vi "ScanSteuerung_to_Datapoints.vi"(2 "Datapoints (-1=estimate)":i32=-1, 3 "ScanSteuerung":T3(array[cluster])=[{"Zeitpunkt [s]"=0.0, "Wirkung"=enum."Abs", "Kanal"=enum."GalvoX", "Wert (/s)"=0.0}, {"Zeitpunkt [s]"=0.0, "Wirkung"=enum."Abs", "Kanal"=enum."GalvoY", "Wert (/s)"=0.5}, {"Zeitpunkt [s]"=0.0, "Wirkung"=enum."LoopStart", "Kanal"=enum."Loop", "Wert (/s)"=3.0}, {"Zeitpunkt [s]"=0.0, "Wirkung"=enum."LoopStart", "Kanal"=enum."Loop", "Wert (/s)"=2.0}, {"Zeitpunkt [s]"=0.0, "Wirkung"=enum."Inc", "Kanal"=enum."GalvoX", "Wert (/s)"=10.0}, {"Zeitpunkt [s]"=0.0, "Wirkung"=enum."IncInc", "Kanal"=enum."GalvoX", "Wert (/s)"=-100.0}, {"Zeitpunkt [s]"=0.0, "Wirkung"=enum."IncInc", "Kanal"=enum."GalvoY", "Wert (/s)"=-100.0}, {"Zeitpunkt [s]"=0.1, "Wirkung"=enum."IncInc", "Kanal"=enum."GalvoY", "Wert (/s)"=100.0}, {"Zeitpunkt [s]"=0.2, "Wirkung"=enum."IncInc", "Kanal"=enum."GalvoX", "Wert (/s)"=100.0}, {"Zeitpunkt [s]"=0.3, "Wirkung"=enum."IncInc", "Kanal"=enum."GalvoY", "Wert (/s)"=-100.0}, {"Zeitpunkt [s]"=0.4, "Wirkung"=enum."IncInc", "Kanal"=enum."GalvoX", "Wert (/s)"=0.0}, {"Zeitpunkt [s]"=0.4, "Wirkung"=enum."LoopEnd", "Kanal"=enum."Loop", "Wert (/s)"=0.0}, {"Zeitpunkt [s]"=0.802, "Wirkung"=enum."LoopEnd", "Kanal"=enum."Loop", "Wert (/s)"=0.0}, {"Zeitpunkt [s]"=2.5, "Wirkung"=enum."IncInc", "Kanal"=enum."GalvoX", "Wert (/s)"=0.0}], 4 "Aktiv":T2(array[ring])=[enum."GalvoX", enum."GalvoY"], 5 "Neues Zeitraster":dbl=1e-05) -> (0 "ScanSteuerungOut":T1(array[cluster])=[{"Zeitpunkt [s]"=0.0, "Wirkung"=enum."Abs", "Kanal"=0.0, "Wert (/s)"=0.0}, {"Zeitpunkt [s]"=0.0, "Wirkung"=enum."Inc", "Kanal"=0.0, "Wert (/s)"=0.0001}, {"Zeitpunkt [s]"=0.0, "Wirkung"=enum."Abs", "Kanal"=1.0, "Wert (/s)"=0.5}, {"Zeitpunkt [s]"=0.0, "Wirkung"=enum."IncInc", "Kanal"=0.0, "Wert (/s)"=-1.0000000000000002e-08}, {"Zeitpunkt [s]"=0.0, "Wirkung"=enum."IncInc", "Kanal"=1.0, "Wert (/s)"=-1.0000000000000002e-08}, {"Zeitpunkt [s]"=10000.0, "Wirkung"=enum."IncInc", "Kanal"=1.0, "Wert (/s)"=1.0000000000000002e-08}, {"Zeitpunkt [s]"=20000.0, "Wirkung"=enum."IncInc", "Kanal"=0.0, "Wert (/s)"=1.0000000000000002e-08}, {"Zeitpunkt [s]"=29999.999999999996, "Wirkung"=enum."IncInc", "Kanal"=1.0, "Wert (/s)"=-1.0000000000000002e-08}, {"Zeitpunkt [s]"=40000.0, "Wirkung"=enum."IncInc", "Kanal"=0.0, "Wert (/s)"=0.0}], 1 "Waveform Graph":dbl[][](graph))   [LabVIEW 2011]
panel:
  out "Datapoints":i32=40001
  out "XY Graph":cluster{dbl[], dbl[]}(graph)
  # "After the loop there has to be at lest one datapoint in one activ channel\nOrder: add abs and rel-values, generate pint, add inc, add incinc to inc\ne.g. at t there is inc: t+1 there is the second pont (t,t+1) with one inc!"
  # "now with incinc support!\nnow with nested loops support!"
  # "Missing error handling for wrong loops!"
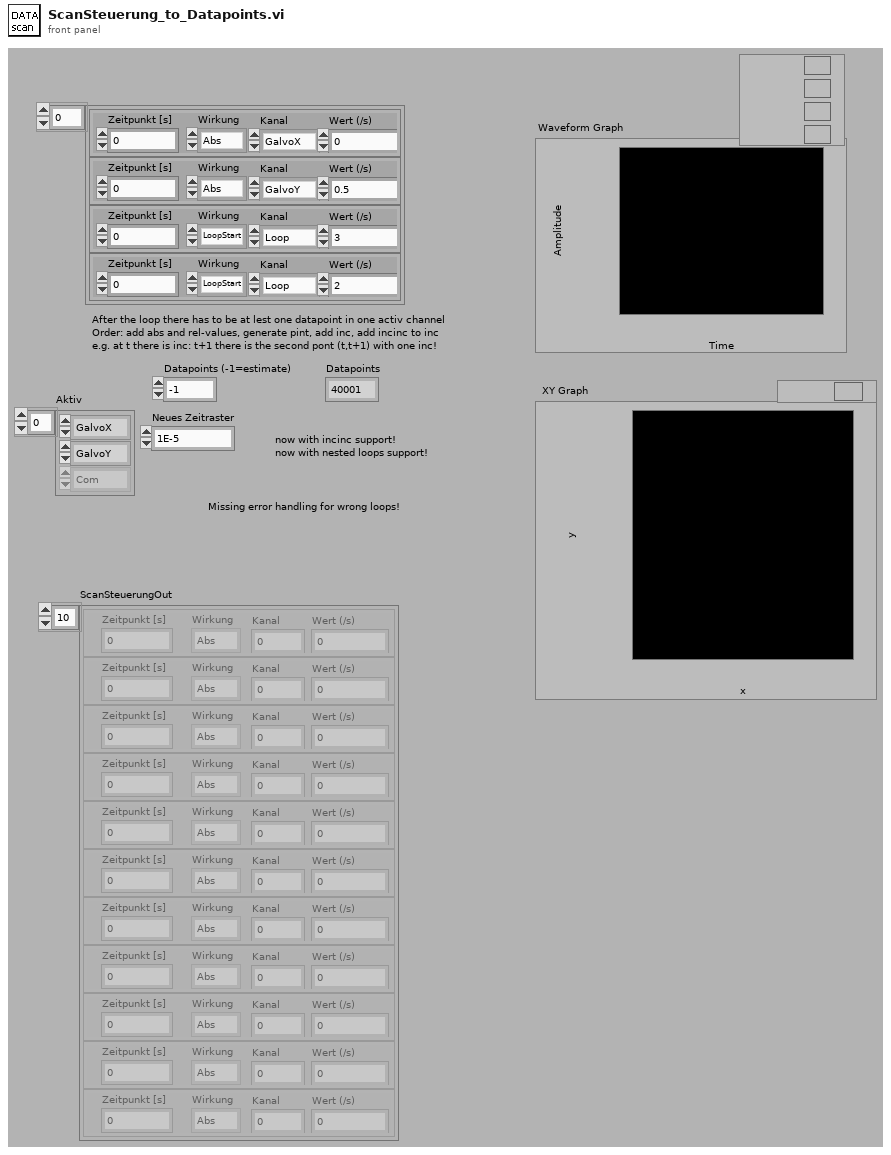
[diagram p1: front panel]
types:
  T1 = cluster{"Zeitpunkt [s]":dbl, "Wirkung":enum16{"Abs", "Rel", "Inc", "IncInc", "LoopStart", "LoopEnd"}, "Kanal":dbl, "Wert (/s)":dbl}[]
  T2 = enum16{"Com", "AnalogConfig", "AnalogValue", "GalvoX", "GalvoY", "Galvo3", "Galvo4", "Digital", "Free", "Loop", "SMoveTime", "Image1X", "Image1Y", "Image2X", "Image2Y"}[]
  T3 = cluster{"Zeitpunkt [s]":dbl, "Wirkung":enum16{"Abs", "Rel", "Inc", "IncInc", "LoopStart", "LoopEnd"}, "Kanal":enum16{"Com", "AnalogConfig", "AnalogValue", "GalvoX", "GalvoY", "Galvo3", "Galvo4", "Digital", "Free", "Loop", "SMoveTime", "Image1X", "Image1Y", "Image2X", "Image2Y"}, "Wert (/s)":dbl}[]
  T4 = cluster{"Time offsets":i32[], "Array":cluster{"Loopstart#":u32, "Loops to do":i32}[]}
  T5 = typedef "ScanControl.ctl" = cluster{"Time [s]":dbl, "action":T6, "channel":T7, "value (/s)":dbl}[]
  T6 = typedef "ScanControl_Action.ctl" = enum16{"Abs", "Rel", "Inc", "IncInc", "LoopStart", "LoopEnd", "WaitTriggerRising"}
  T7 = typedef "ScanControl_Channel.ctl" = enum16{"Com", "AnalogConfig", "AnalogValue", "GalvoX", "GalvoY", "Galvo3", "Galvo4", "Digital", "Free", "Loop", "SMoveTime", "Image1X", "Image1Y", "Image2X", "Image2Y"}
  T8 = cluster{"Zeitpunkt [s]":dbl, "Wirkung":enum16{"Abs", "Rel", "Inc", "IncInc", "LoopStart", "LoopEnd"}, "Kanal":i32, "Wert (/s)":dbl}[]
  T9 = cluster{"Zeitpunkt [s]":dbl, "Wirkung":enum16{"Abs", "Rel", "Inc", "IncInc", "LoopStart", "LoopEnd"}, "Kanal":i32, "Wert (/s)":dbl}
  T10 = enum16{"Abs", "Rel", "Inc", "IncInc", "LoopStart", "LoopEnd"}
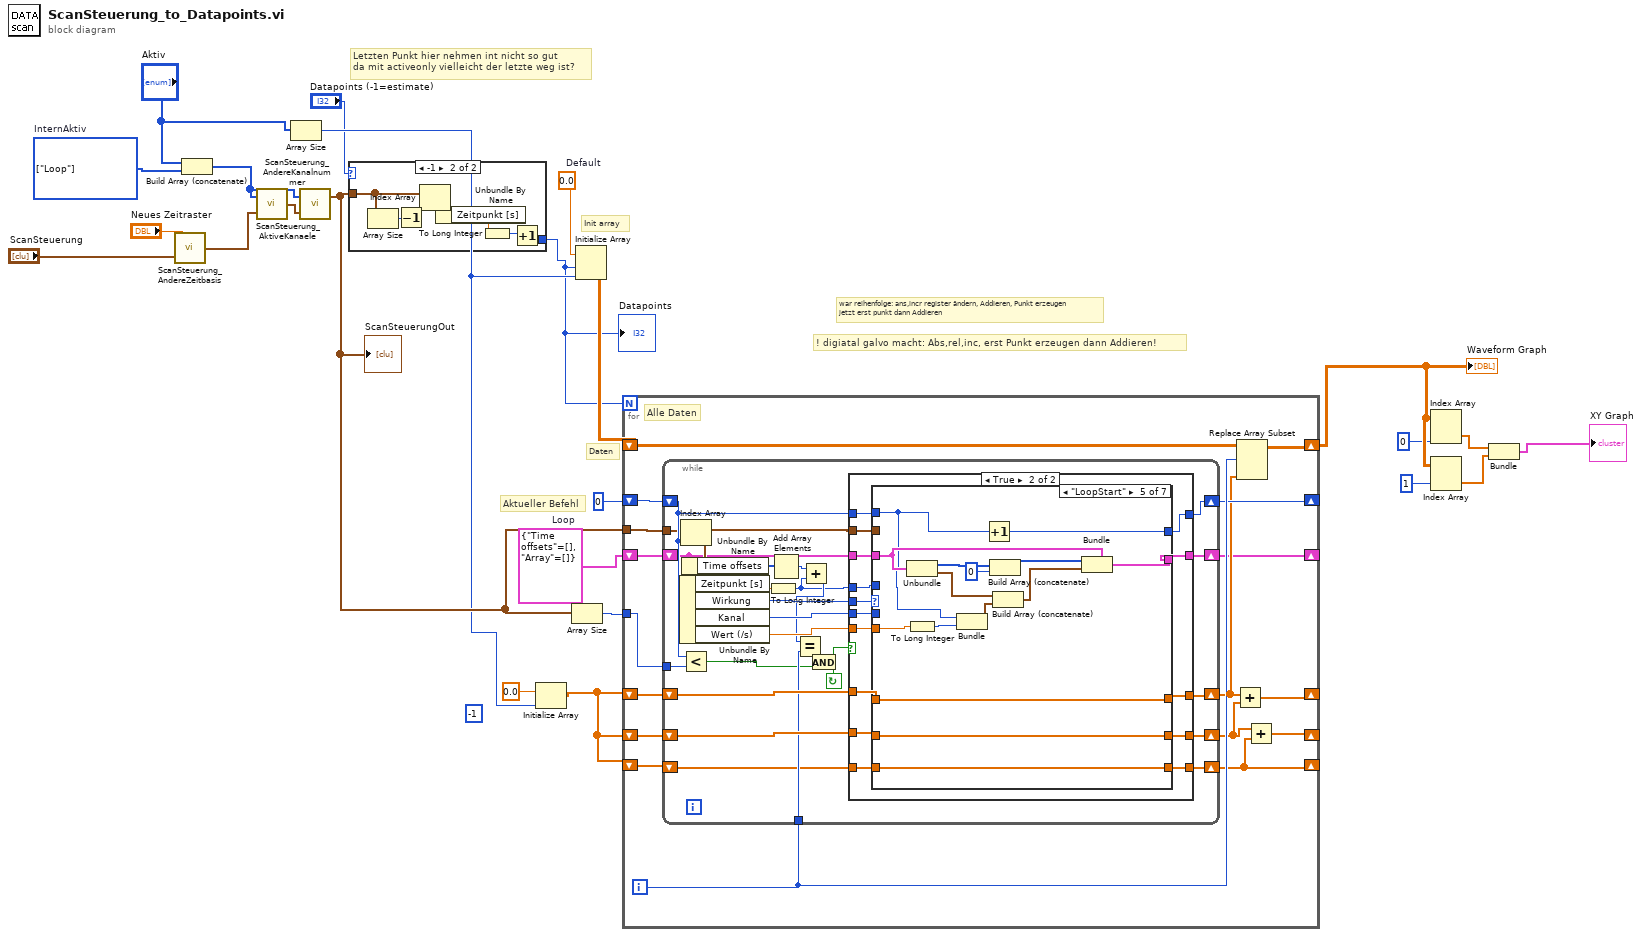
[diagram p0: block diagram]
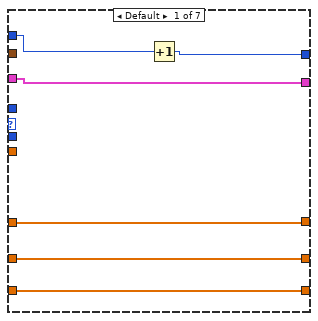
[diagram p4: hidden frame]
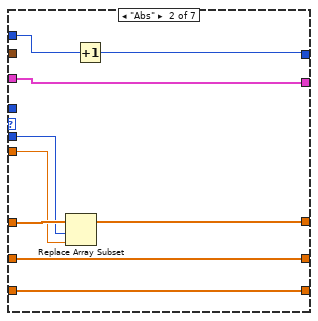
[diagram p5: hidden frame]
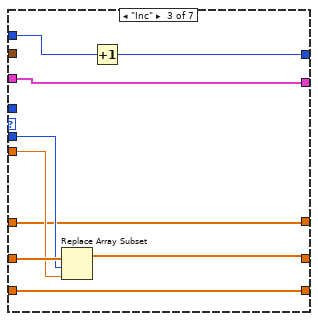
[diagram p6: hidden frame]
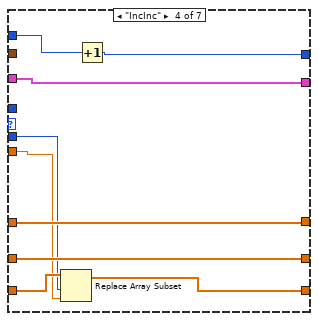
[diagram p7: hidden frame]
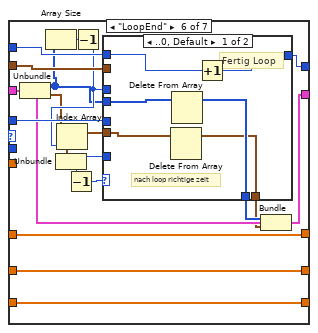
[diagram p8: hidden frame]
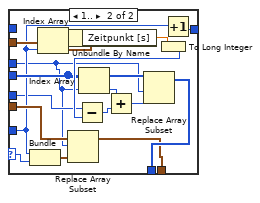
[diagram p9: hidden frame]
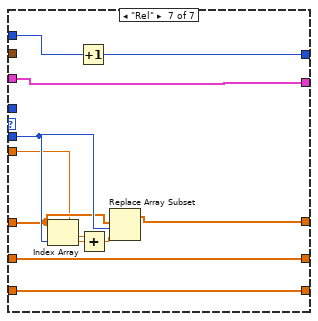
[diagram p10: hidden frame]
diagram:
  (unwired) -1 ("LoopLevel")
  w1 = T4 {"Time offsets"=[], "Array"=[]}  # Loop
  w17 = T2 [enum."Loop"] items=["Com", "AnalogConfig", "AnalogValue", "GalvoX", "GalvoY", "Galvo3", "Galvo4", "Digital", "Free", "Loop", "SMoveTime", "Image1X", "Image1Y", "Image2X", "Image2Y"]  # InternAktiv
  w24 = 0.0  # Default
  # "! digiatal galvo macht: Abs,rel,inc, erst Punkt erzeugen dann Addieren!"
  # "war reihenfolge: ans,incr register ändern, Addieren, Punkt erzeugen\njetzt erst punkt dann Addieren"
  # "Letzten Punkt hier nehmen int nicht so gut\nda mit activeonly vielleicht der letzte weg ist?"
  # "Aktueller Befehl"
  # "Daten"
  # "Init array"
  n1 = call "ScanSteuerung_AndereZeitbasis.vi"("ScanSteuerung"="ScanSteuerung", "Neues Zeitraster"="Neues Zeitraster") -> ("ScanSteuerungOut"=w13:T5)
  n2 = Build Array (concatenate)("Aktiv", w17) -> (w15:T2)
  n3 = call "ScanSteuerung_AktiveKanaele.vi"("ScanSteuerung"=w13, "Aktiv"=w15) -> ("ScanSteuerungOut"=w19:T5)
  n4 = Array Size(array="Aktiv") -> (size(s)=w14:i32)
  n5 = call "ScanSteuerung_AndereKanalnummer.vi"("ScanSteuerung"=w19, "Neue Kanalnummer (nicht gefunden gibt 0!)"=w15) -> ("ScanSteuerungOut"=w18:T8)  [unwired: 1 out]
  "ScanSteuerungOut" <- w18
  n6 = case shown="-1" "Datapoints (-1=estimate)" {
    selector: "Datapoints (-1=estimate)" -> [w25 _]
    tunnel: w18 -> [_ w28]
    tunnel: [w25 w26] -> w4
    frame 0, Default {
    }
    frame -1 {
      n7 = Array Size(array=w28) -> (size(s)=w32:i32)
      n8 = Decrement(x=w32) -> (x-1=w31:i32)
      n9 = Index Array(array=w28, index=w31) -> (element=w30:T9)
      n10 = Unbundle By Name(w30) -> ("Zeitpunkt [s]"=w29:dbl)
      n11 = To Long Integer(number=w29) -> (32bit integer=w27:i32)
      n12 = Increment(x=w27) -> (x+1=w26:i32)
    }
  }
  "Datapoints" <- w4
  n13 = Initialize Array(0.0 ("element"), w14) -> (w2:dbl[])
  n14 = Array Size(array=w18) -> (size(s)=w21:i32)
  n15 = Initialize Array(w24, w4, w14) -> (w22:dbl[][])
  n16 = for {
    N: w4 -> [_]
    shift-left: w2 -> [w47]
    shift-right: [w43] -> _
    tunnel: w21 -> [w40]
    shift-left: u32 0 -> [w48]
    shift-right: [w41] -> _
    shift-left: w22 -> [w45]
    shift-right: [w44] -> w11
    tunnel: w18 -> [w49]
    shift-right: [w37] -> _
    shift-left: w2 -> [w46]
    shift-right: [w35] -> _
    shift-left: w2 -> [w38]
    shift-right: [w33] -> _
    shift-left: w1 -> [w34]
    i -> [w42]
    # "Alle Daten"
    n17 = while {
      tunnel: w49 -> [w54]
      shift-right: [w66] -> w41
      shift-left: w48 -> [w61]
      shift-right: [w69] -> w39
      shift-left: w47 -> [w73]
      shift-right: [w68] -> w36
      shift-left: w46 -> [w72]
      tunnel: w42 -> [w65]
      tunnel: w40 -> [w60]
      shift-right: [w55] -> w35
      shift-left: w38 -> [w56]
      shift-right: [w52] -> w33
      shift-left: w34 -> [w53]
      stop <- w57 continue-if-true
      n18 = Index Array(array=w54, index=w61) -> (element=w74:T9)
      n19 = Unbundle By Name(w74) -> ("Zeitpunkt [s]"=w63:dbl, "Wirkung"=w67:T10, "Kanal"=w71:i32, "Wert (/s)"=w70:dbl)
      n20 = Less?(x=w61, y=w60) -> (x < y?=w58:bool)
      n21 = Unbundle By Name(w53) -> ("Time offsets"=w51:i32[])
      n22 = To Long Integer(number=w63) -> (32bit integer=w62:i32)
      n23 = Add Array Elements(numeric array=w51) -> (sum=w50:i32)
      n24 = Add(x=w50, y=w62) -> (x+y=w64:i32)
      n25 = Equal?(x=w64, y=w65) -> (x = y?=w59:bool)
      n26 = And(x=w59, y=w58) -> (x .and. y?=w57:bool)
      n27 = case shown="True" w57 {
        tunnel: w73 -> [w79 w94]
        tunnel: w72 -> [w78 w93]
        tunnel: w71 -> [_ w92]
        tunnel: w70 -> [_ w91]
        tunnel: [w79 w90] -> w69
        tunnel: [w78 w89] -> w68
        tunnel: w67 -> [_ w88]
        tunnel: w61 -> [w77 w87]
        tunnel: [w77 w86] -> w66
        tunnel: w62 -> [_ w85]
        tunnel: w56 -> [w76 w84]
        tunnel: [w76 w83] -> w55
        tunnel: w54 -> [_ w82]
        tunnel: w53 -> [w75 w81]
        tunnel: [w75 w80] -> w52
        frame False {
          # "Fertig"
        }
        frame True {
          n28 = case shown="\"LoopStart\"" w88 {
            tunnel: w94 -> [w98 w109 w114 w127 w142 w161 w192]
            tunnel: w93 -> [w97 w105 w118 w126 w141 w160 w191]
            tunnel: w92 -> [_ w108 w116 w122 _ _ w193]
            tunnel: w91 -> [_ w107 w115 w121 w140 _ w190]
            tunnel: [w98 w106 w114 w127 w142 w161 w195] -> w90
            tunnel: [w97 w105 w117 w126 w141 w160 w191] -> w89
            tunnel: w87 -> [w100 w104 w113 w125 w135 w158 w188]
            tunnel: [w95 w103 w112 w124 w139 w159 w187] -> w86
            tunnel: w85 -> [_ _ _ _ _ w157 _]
            tunnel: w84 -> [w96 w102 w111 w123 w138 w156 w186]
            tunnel: [w96 w102 w111 w120 w138 w156 w186] -> w83
            tunnel: w82 -> [_ _ _ _ _ w155 _]
            tunnel: w81 -> [w99 w101 w110 w119 w136 w151 w185]
            tunnel: [w99 w101 w110 w119 w137 w152 w185] -> w80
            frame Default {
              n29 = Increment(x=w100) -> (x+1=w95:u32)
            }
            frame "Abs" {
              n30 = Replace Array Subset(array=w109, new element=w107, index=w108) -> (w106:dbl[])
              n31 = Increment(x=w104) -> (x+1=w103:u32)
            }
            frame "Inc" {
              n32 = Replace Array Subset(array=w118, new element=w115, index=w116) -> (w117:dbl[])
              n33 = Increment(x=w113) -> (x+1=w112:u32)
            }
            frame "IncInc" {
              n34 = Replace Array Subset(array=w123, new element=w121, index=w122) -> (w120:dbl[])
              n35 = Increment(x=w125) -> (x+1=w124:u32)
            }
            frame "LoopStart" {
              n36 = Unbundle(w136) -> ("Time offsets"=w129:i32[], "Array"=w128:cluster{"Loopstart#":u32, "Loops to do":i32}[])
              n37 = To Long Integer(number=w140) -> (32bit integer=w134:i32)
              n38 = Bundle(w135, w134) -> (w132:cluster{u32, i32})  [unwired: 1 out]
              n39 = Increment(x=w135) -> (x+1=w139:u32)
              n40 = Build Array (concatenate)(w129, 0) -> (w131:i32[])
              n41 = Build Array (concatenate)(w128, w132) -> (w133:cluster{"Loopstart#":u32, "Loops to do":i32}[])
              n42 = Bundle(cluster=w136, "Time offsets"=w131, "Array"=w133) -> (w137:T4)
            }
            frame "LoopEnd" {
              n43 = Unbundle(w151) -> ("Time offsets"=w144:i32[], "Array"=w143:cluster{"Loopstart#":u32, "Loops to do":i32}[])
              n44 = Array Size(array=w144) -> (size(s)=w146:i32)
              n45 = Decrement(x=w146) -> (x-1=w145:i32)
              n46 = Index Array(array=w143, index=w145) -> (element=w150:cluster{"Loopstart#":u32, "Loops to do":i32})
              n47 = Unbundle(w150) -> ("Loopstart#"=w153:u32, "Loops to do"=w154:i32)
              n48 = Decrement(x=w154) -> (x-1=w149:i32)
              n49 = case shown="..0, Default" w149 {
                selector: w149 -> [_ w171]
                tunnel: w144 -> [w165 w175]
                tunnel: [w166 w184] -> w159
                tunnel: w158 -> [w167 _]
                tunnel: w157 -> [_ w169]
                tunnel: w155 -> [_ w182]
                tunnel: w153 -> [_ w170]
                tunnel: w145 -> [_ w168]
                tunnel: [w164 w176] -> w148
                tunnel: w143 -> [w163 w173]
                tunnel: [w162 w174] -> w147
                frame ..0, Default {
                  # "nach loop richtige zeit"
                  # "Fertig Loop"
                  n50 = Delete From Array(array=w163) -> (array with subset deleted=w162:cluster{"Loopstart#":u32, "Loops to do":i32}[])  [unwired: 2 in, 1 out]
                  n51 = Delete From Array(array=w165) -> (array with subset deleted=w164:i32[])  [unwired: 2 in, 1 out]
                  n52 = Increment(x=w167) -> (x+1=w166:u32)
                }
                frame 1.. {
                  n53 = Bundle("Loopstart#"=w170, w171) -> (w172:cluster{"Loopstart#":u32, i32})  [unwired: 1 out]
                  n54 = Index Array(array=w182, index=w170) -> (element=w181:T9)
                  n55 = Unbundle By Name(w181) -> ("Zeitpunkt [s]"=w180:dbl)
                  n56 = Replace Array Subset(array=w173, new element=w172, index=w168) -> (w174:cluster{"Loopstart#":u32, "Loops to do":i32}[])
                  n57 = Index Array(array=w175, index=w168) -> (element=w178:i32)
                  n58 = To Long Integer(number=w180) -> (32bit integer=w179:i32)
                  n59 = Subtract(x=w169, y=w179) -> (x-y=w183:i32)
                  n60 = Add(x=w178, y=w183) -> (x+y=w177:i32)
                  n61 = Replace Array Subset(array=w175, new element=w177, index=w168) -> (w176:i32[])
                  n62 = Increment(x=w170) -> (x+1=w184:u32)
                }
              }
              n63 = Bundle(cluster=w151, "Time offsets"=w148, "Array"=w147) -> (w152:T4)
            }
            frame "Rel" {
              n64 = Index Array(array=w192, index=w193) -> (element=w189:dbl)
              n65 = Increment(x=w188) -> (x+1=w187:u32)
              n66 = Add(x=w190, y=w189) -> (x+y=w194:dbl)
              n67 = Replace Array Subset(array=w192, new element=w194, index=w193) -> (w195:dbl[])
            }
          }
        }
      }
    }
    n68 = Add(x=w39, y=w36) -> (x+y=w43:dbl[])
    n69 = Replace Array Subset(array=w45, new element=w39, index (row)=w42) -> (w44:dbl[][])  [unwired: 1 in]
    n70 = Add(x=w36, y=w35) -> (x+y=w37:dbl[])
  }
  "Waveform Graph" <- w11
  n71 = Index Array(array=w11, index (col)=0) -> (element=w10:dbl[])  [unwired: 1 in]
  n72 = Index Array(array=w11, index (col)=1) -> (element=w9:dbl[])  [unwired: 1 in]
  n73 = Bundle(w10, w9) -> (→"XY Graph":cluster{dbl[], dbl[]})  [unwired: 1 out]
